vi "Get DLL version.vi"() -> (0 "Error":errorcluster, 1 "DLL path":path, 2 "DLL version":string)   [LabVIEW 2018]
uses:
  Coherent global.vi
panel:
  # "PN 06/11/2014\n      08/04/2019"
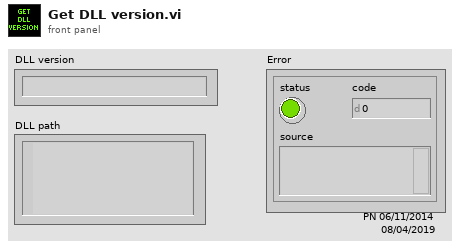
[diagram p1: front panel]
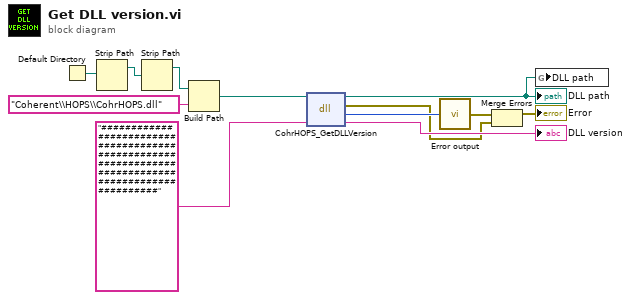
[diagram p0: block diagram]
diagram:
  n1 = Default Directory() -> (w6:path)
  n2 = Strip Path(path=w6) -> (stripped path=w5:path)  [unwired: 1 out]
  n3 = Strip Path(path=w5) -> (stripped path=w4:path)  [unwired: 1 out]
  n4 = Build Path(base path=w4, name or relative path="Coherent\\HOPS\\CohrHOPS.dll") -> (appended path=w8:path)
  n5 = dll-call lib="?" fn="CohrHOPS_GetDLLVersion"(path in=w8, "version"="####################################################################################################" ("headType")) -> (path out=w7:path, error out=w3:errorcluster, "return value"=w11:i32, "version"=→"DLL version":string)  [unwired: 2 in]
  "DLL path" <- w7
  n6 = call "Error output.vi"("I32 err code"=w11) -> ("Error Out"=w2:errorcluster)
  n7 = Merge Errors(w2, w3) -> (→"Error":errorcluster)
  n8 = global write "Coherent global.vi" "DLL path"(w7) -> ()
